vi "Main_01a.vi"() -> ()   [LabVIEW 2024]
panel:
  out "Right List":i32[](array[numeric])
  out "Left List":i32[](array[numeric])
  out "Answer 2344935":i32
  in  "Puzzle":string="80421   40193\n69841   31045\n47850   64065\n63141   52072\n32908   83033\n33395   25559\n78513   59127\n91270   76329\n65508   34159\n27139   15788\n13228   50396\n43186   29116\n55392   52441\n19309   68909\n72798   54258\n31590   11220\n32125   81946\n58099   50396\n16614   76682\n60604   12184\n21251   26105\n56053   96112\n47903   13396\n72956   11681\n66315   11220\n54499   96112\n38390   83884\n69211   52732\n69235   52441\n83831   49092\n25782   75523\n35417   15162\n45889   82918\n76191   97182\n95942   49643\n30121   83884\n86470   16217\n23572   11220\n69703   80739\n45792   21543\n76682   70230\n79585   83884\n64501   69361\n55546   92076\n43632   87826\n93309   17223\n73996   69071\n83466   42385\n73963   19398\n36643   98070\n43789   15788\n54302   70897\n83362   50227\n60881   66983\n61881   17864\n81520   52171\n99147   41180\n63427   16217\n50290   40193\n19315   20520\n84997   27666\n45495   40509\n81512   76682\n93459   11220\n28126   72353\n38227   11681\n49613   27677\n26858   40193\n16759   51946\n42145   90200\n64421   88733\n97361   16019\n32616   75596\n30875   90149\n82019   50759\n90554   83033\n42030   75763\n64459   32394\n45152   83884\n51375   48768\n71487   93793\n69694   84439\n97213   70998\n65471   90900\n69237   48307\n50672   58376\n61500   58064\n22831   76682\n63626   90356\n43195   87826\n67468   11770\n59753   97698\n34386   97698\n84851   23296\n96001   69910\n41418   13027\n82815   27666\n37012   17864\n45122   57830\n81552   44943\n18717   33011\n28726   87826\n29453   52441\n82398   24963\n47384   87826\n24205   50966\n80001   43568\n17033   21145\n74890   54233\n59065   58047\n33505   96112\n96403   34213\n35992   94345\n74353   27666\n59539   37101\n90355   71860\n86007   11220\n50733   76682\n75113   94664\n56735   87038\n27654   16492\n39478   47633\n70998   95331\n19885   38941\n47463   26105\n74771   28343\n56762   87773\n89980   35218\n35434   71473\n97275   53382\n97389   28343\n55060   11220\n83189   74164\n65464   75140\n15091   58376\n49752   94345\n55978   50227\n13991   40193\n58778   69071\n99285   16217\n37693   40193\n61282   71473\n34624   87374\n53881   13912\n67666   58376\n51235   52441\n80739   99593\n40193   97698\n94214   83205\n13145   72473\n88888   40193\n46957   96567\n92406   59738\n85389   13942\n55969   52441\n91426   46497\n92608   63775\n71473   24823\n51744   50396\n77645   42696\n34121   96112\n99775   96112\n89480   98660\n42647   95861\n35131   98522\n22031   76805\n10282   43806\n82323   65743\n79408   89179\n50692   85420\n89878   70998\n46431   17223\n99643   52441\n61276   68075\n14058   83884\n94292   17411\n92506   40193\n91012   17223\n51557   55254\n50846   96567\n20336   84821\n71617   81946\n40314   84439\n42990   89703\n62455   27446\n65790   94345\n57568   65105\n13052   79090\n30028   96128\n42028   58852\n47372   87826\n44459   90200\n67988   66776\n28313   84439\n52545   94345\n17108   37412\n16113   11681\n56064   54165\n60025   37314\n85545   11681\n68437   25575\n46677   20626\n53308   28343\n79483   70998\n54308   55727\n26755   69337\n73791   50227\n33565   83884\n35359   17223\n47840   26266\n50109   75074\n88842   39316\n84439   97698\n86029   96112\n39964   79122\n37828   69071\n73120   96567\n67688   50227\n61996   70230\n62643   82883\n99604   28343\n18054   76682\n52441   97698\n45131   58376\n32102   53380\n60963   53418\n73803   41652\n56361   70998\n74041   77517\n14940   84439\n80439   26105\n79199   83033\n41700   83033\n35229   65677\n64958   84439\n51246   78550\n23506   31244\n26237   40038\n49105   27712\n62117   37779\n76884   94345\n56414   62009\n88424   80739\n97192   15788\n70374   59226\n53515   76682\n85931   28343\n50925   38390\n51959   96567\n98082   28525\n37588   29342\n52624   37871\n28331   16217\n73762   94345\n73815   38390\n38573   25210\n88916   97698\n66917   28343\n47055   73500\n97902   34391\n16580   82128\n18015   91780\n77218   14792\n22251   37702\n62344   94345\n49811   73150\n43220   58572\n93889   76682\n70259   90173\n16985   26105\n93371   50227\n93434   49229\n97412   55737\n69071   39598\n70682   90271\n31536   30421\n81650   96112\n66094   70998\n94447   83052\n70230   87681\n69613   93387\n50227   85660\n32751   83903\n12441   41367\n64171   79090\n88431   75578\n33033   96567\n96305   79090\n17193   52441\n42766   27666\n30798   50396\n18160   14792\n86048   69517\n26894   10883\n72243   38390\n48910   96875\n80507   90612\n77344   83033\n11713   96112\n36810   50227\n91347   11220\n20755   76682\n50353   95421\n63754   63013\n22119   25388\n35010   38390\n39083   90678\n16379   13640\n47651   67154\n50798   71473\n64108   83884\n62368   85420\n87732   54461\n44496   74078\n50396   16217\n32142   94345\n12969   50227\n63851   24208\n59124   89844\n24929   21174\n55229   84439\n78807   15788\n58298   50396\n16926   96567\n83884   50396\n63542   49739\n76625   41626\n97382   32976\n40464   38390\n14575   10840\n63334   71473\n25579   40921\n71524   96567\n50616   93389\n81504   17864\n10618   32838\n65653   11681\n74217   76682\n17739   45245\n12975   56728\n92629   12987\n13610   68591\n24487   83033\n12475   81946\n31651   39134\n32359   81946\n41174   79359\n63548   65603\n55031   50396\n59183   58376\n74036   69252\n33977   71473\n39977   40407\n32033   40193\n90147   83033\n23940   30137\n67597   33156\n64295   99755\n72689   96112\n92379   83884\n59904   17864\n59250   54829\n31693   34134\n88853   97698\n46754   31254\n58208   11220\n98626   11220\n46741   70998\n36408   63013\n18581   87826\n63114   28343\n97394   81946\n93270   97698\n80744   59372\n97689   57651\n87482   58376\n11896   75807\n65025   96196\n15892   54686\n68939   24270\n16022   53606\n36023   85420\n95998   43637\n61265   38390\n79090   11220\n81946   99814\n63895   78782\n83527   90200\n51915   62980\n22548   20223\n58376   26608\n81705   24971\n99116   26106\n92178   77949\n98976   38390\n81016   28343\n52646   79090\n29911   88246\n23834   92181\n46484   89669\n68488   44503\n74484   29808\n89780   86262\n96112   75203\n51392   42994\n19800   23307\n49890   41317\n98098   94345\n57894   69730\n59120   93793\n86825   83884\n41981   84710\n69860   70998\n25576   35489\n42850   23083\n34439   85430\n91153   35450\n59806   16217\n87651   74318\n15466   76682\n94237   22001\n45392   47159\n35295   95111\n86122   88173\n28631   50396\n34798   26613\n61839   13468\n61723   96112\n14034   96112\n30006   16217\n14649   26145\n86294   80739\n32258   11681\n92857   50396\n86334   58376\n10895   84439\n63194   85936\n76887   96027\n68733   26105\n41207   63013\n28365   88512\n24732   38390\n67548   49710\n81155   48747\n41815   96112\n51642   69071\n62718   81572\n59606   98715\n74964   13588\n64466   17223\n96982   46340\n84527   94623\n69698   11220\n11144   23375\n57947   97698\n41007   80545\n11681   32334\n94807   43967\n54555   94345\n16363   93419\n65623   45980\n42388   45727\n48482   79090\n85324   81581\n59768   37611\n62042   11681\n90240   19425\n66983   24278\n98892   42679\n35839   35139\n17825   39236\n74183   28343\n94347   48434\n82766   84797\n12488   62200\n11529   58265\n82862   27666\n63390   87826\n87638   60767\n69964   71473\n94668   76682\n58958   52441\n75722   97743\n68139   11220\n58242   75810\n92586   40193\n29680   94345\n33347   73583\n74149   73747\n88092   94345\n82865   45901\n88894   38390\n40872   97309\n85420   93793\n80641   69071\n57680   79788\n50575   63583\n45838   28855\n77834   63196\n36094   58852\n93487   19648\n98316   79122\n89283   97494\n81283   78824\n78086   84439\n70708   27959\n64643   44369\n39933   56445\n68663   28343\n97698   10803\n79122   51608\n35053   96112\n88445   87826\n59362   81946\n58091   67264\n48218   93793\n64495   16994\n38395   71473\n61884   50396\n84809   84439\n90363   78607\n39707   76682\n66866   83033\n76807   80277\n98492   83033\n65436   84059\n69199   68798\n62230   83884\n51938   18013\n99036   22915\n20508   84439\n41393   50396\n47979   58852\n74140   70998\n42029   88646\n43056   14163\n96145   39532\n80632   64382\n56985   85420\n63903   41993\n11220   93712\n94345   15788\n43760   56901\n93453   58852\n35914   74746\n73054   44762\n45629   40193\n77231   55896\n77041   38390\n96658   74157\n46466   17606\n88020   77476\n51115   61806\n24234   81946\n17382   79090\n38939   78416\n55399   95124\n74933   97972\n17223   11832\n20126   25792\n84054   91443\n84057   96112\n88765   83033\n27933   54577\n48695   78824\n90200   51999\n74599   38503\n61441   90200\n66742   38390\n23353   26105\n37362   82425\n38602   44514\n41407   71473\n51001   62633\n98321   40630\n75078   11681\n68245   24288\n49051   14363\n36869   25312\n17659   47253\n74211   69071\n41285   22997\n89913   71473\n35951   34861\n67158   50396\n43938   15553\n72373   24972\n40926   97698\n63013   85420\n19477   71473\n79722   19841\n28842   83920\n14541   55730\n31500   75763\n51488   32218\n18889   96567\n57241   17864\n51819   47021\n21973   30568\n13743   10104\n87695   43875\n90862   27666\n16780   65150\n24792   58376\n28715   69071\n40287   78011\n59897   84439\n16124   83884\n34237   44208\n80709   83186\n12989   55204\n96071   63816\n78189   63337\n37586   98216\n19413   51370\n64986   70521\n93855   48927\n57998   25233\n42676   58360\n93905   29575\n18012   58243\n28846   54313\n97083   50396\n59982   20815\n95409   88260\n57482   70230\n69515   83884\n78295   69071\n72645   71473\n71966   28343\n98274   84439\n34068   28343\n96135   40193\n65836   15788\n23264   84439\n19621   51691\n75945   40091\n29573   47799\n14879   79090\n28207   38390\n11483   15774\n32877   80739\n36254   96567\n65116   27258\n14250   93650\n23902   96112\n89984   35958\n82242   33004\n12762   62900\n81194   99347\n72193   37712\n71644   74162\n46588   52441\n27739   70311\n35648   70998\n44410   87233\n46656   27666\n31914   71473\n90034   78824\n61968   83033\n36567   29131\n78387   67697\n33453   57266\n24915   40540\n70857   52975\n28343   81423\n92106   87378\n56025   82509\n32851   98692\n51436   97147\n70601   71473\n70452   33153\n39288   15788\n17976   11220\n15788   58376\n40113   53779\n25192   88120\n31980   98924\n80317   91384\n67936   10228\n14839   75691\n55689   75265\n28107   90207\n49283   17864\n27666   52539\n26105   26025\n71897   10363\n65171   58095\n87061   76361\n58586   84439\n90319   17223\n12401   11681\n60665   21206\n66454   77367\n58801   69471\n12007   11220\n59620   71043\n14269   33941\n84020   34182\n21849   61119\n19934   93793\n49226   64719\n59477   58376\n67180   38390\n69143   84212\n29611   69071\n74186   73216\n44892   47027\n88341   63662\n93425   27666\n58009   40217\n61426   88678\n14176   17223\n19374   19815\n15924   63644\n31338   90200\n20061   96567\n77739   17223\n39213   79090\n86112   44465\n59347   96112\n52900   88643\n49030   41964\n79160   96112\n60822   33345\n87682   46340\n92223   67780\n75763   68868\n58470   38390\n22344   11681\n60094   70230\n53703   65992\n60348   41120\n14792   81993\n53271   21427\n67055   17864\n64402   49401\n46340   71473\n67425   80739\n33676   91364\n20261   93934\n33464   45079\n47333   87047\n99552   33828\n46700   29241\n34066   38390\n63635   81946\n64943   90200\n93222   70855\n39852   27666\n54215   27846\n91837   81435\n13206   92486\n34097   89083\n67571   63013\n65552   28794\n93206   16217\n57258   46746\n12355   95783\n45193   39825\n78824   41374\n79640   28343\n33304   46968\n52405   53684\n80165   79090\n63764   98552\n50867   62235\n55169   67322\n17385   63412\n93847   84439\n86220   96567\n56922   26105\n93793   70998\n46061   15119\n60608   50227\n53721   82034\n37048   97113\n78634   17392\n16149   11220\n96567   17864\n67761   15242\n43531   45273\n28649   81808\n16807   11681\n35016   38390\n36328   15788\n47350   87826\n83703   76682\n96035   68596\n89445   40193\n39175   22115\n46972   69071\n86512   64757\n70145   30941\n92472   94345\n28607   84439\n97839   80739\n46293   22854\n39471   56487\n40895   81224\n79054   15540\n19112   99099\n87456   97698\n64947   93293\n46868   17223\n61194   51103\n94011   51317\n93446   67760\n51603   79090\n98462   32618\n87627   14792\n50434   28343\n80823   87826\n85968   11220\n70582   94611\n69082   69071\n82872   75587\n66992   93001\n16652   81390\n45397   67124\n48288   12534\n16683   60958\n28845   17300\n73108   85770\n10887   14000\n86564   58432\n73753   15788\n58200   60971\n14724   10521\n22429   86503\n15636   73714\n42007   50396\n83033   28343\n11018   17864\n84668   59520\n34407   50227\n21979   66729\n20788   97698\n88249   71473\n29698   76682\n18861   90200\n33097   18831\n84374   38460\n42337   49469\n96184   11220\n93246   50708\n59059   17223\n94799   11681\n94592   90061\n16217   87826\n15119   39287\n98585   71473\n96536   42853\n70453   24363\n98772   69071\n86608   28722\n96532   50396\n29434   83821\n45190   18432\n39085   52441\n14544   27666\n98167   83884\n40247   35796\n58852   95208\n63594   94345\n37166   70696\n37060   97185\n78269   17223\n31684   50764\n17864   52599\n24791   33385\n88009   94208\n44960   66939\n94307   25038\n97941   92450\n84015   83884\n18910   52086\n65496   17223\n40031   34551\n85606   91632\n61769   76682\n16593   90387\n18746   84938\n37661   78508\n74488   71473\n10696   57789\n73457   33795\n36702   93793\n50523   40193\n54560   97491\n31840   38390\n76940   40193\n16870   11681\n59273   30259\n87826   11069\n42351   47872\n46704   17864\n60979   83884\n13487   66385\n89414   94345\n95781   78824\n81388   50396\n76147   16961\n47912   27666\n38794   15498\n42095   60345\n50754   85082\n47680   11681\n74650   63013\n79979   27666\n93963   91067\n12526   51125\n15421   50227\n14489   17864\n19890   71473\n39148   69071\n35061   43580\n13873   78824\n65002   84439\n44196   70230\n91160   27666\n66243   17864\n68520   52987\n57313   11001\n97451   71232\n45491   88748\n72806   28343\n10935   96112\n26571   50227\n36588   11220\n97082   47405\n74083   76682\n13709   28343\n71565   60347\n67060   89690\n89812   68984\n64357   18200\n13576   86923\n17785   52441\n90523   87826\n48169   84439\n49404   96112\n38548   93793\n10365   50396\n85079   97698\n87583   95586\n63995   97698\n37765   62288\n96507   26105\n74440   19405\n96601   94432\n37066   38390\n42143   11552\n33431   27666\n77502   63356\n33810   52441\n14847   36105\n21823   66983\n57868   71473\n84231   27666\n87717   52441\n53162   97698\n35374   65715\n34570   26105\n20224   36282\n71791   40193\n18833   48330\n12194   83762\n92449   38390\n18772   71473\n59035   57762\n60408   76682\n62373   63013\n79934   40193\n82312   59106\n22944   72620\n15001   50192\n42041   93793\n27226   80739\n68012   30136\n22148   34448\n15624   94345\n79255   39850\n80907   18558\n92896   15318\n25411   94345\n33580   81946\n71575   70650\n47700   79090\n75865   16217\n48756   81946\n98547   75763\n23220   38390\n15241   79090\n18586   33917\n22280   40494\n35998   69327\n60853   95280\n38251   50396\n52525   87826"
  in  "Example":string="3   4\n4   3\n2   5\n1   3\n3   9\n3   3"
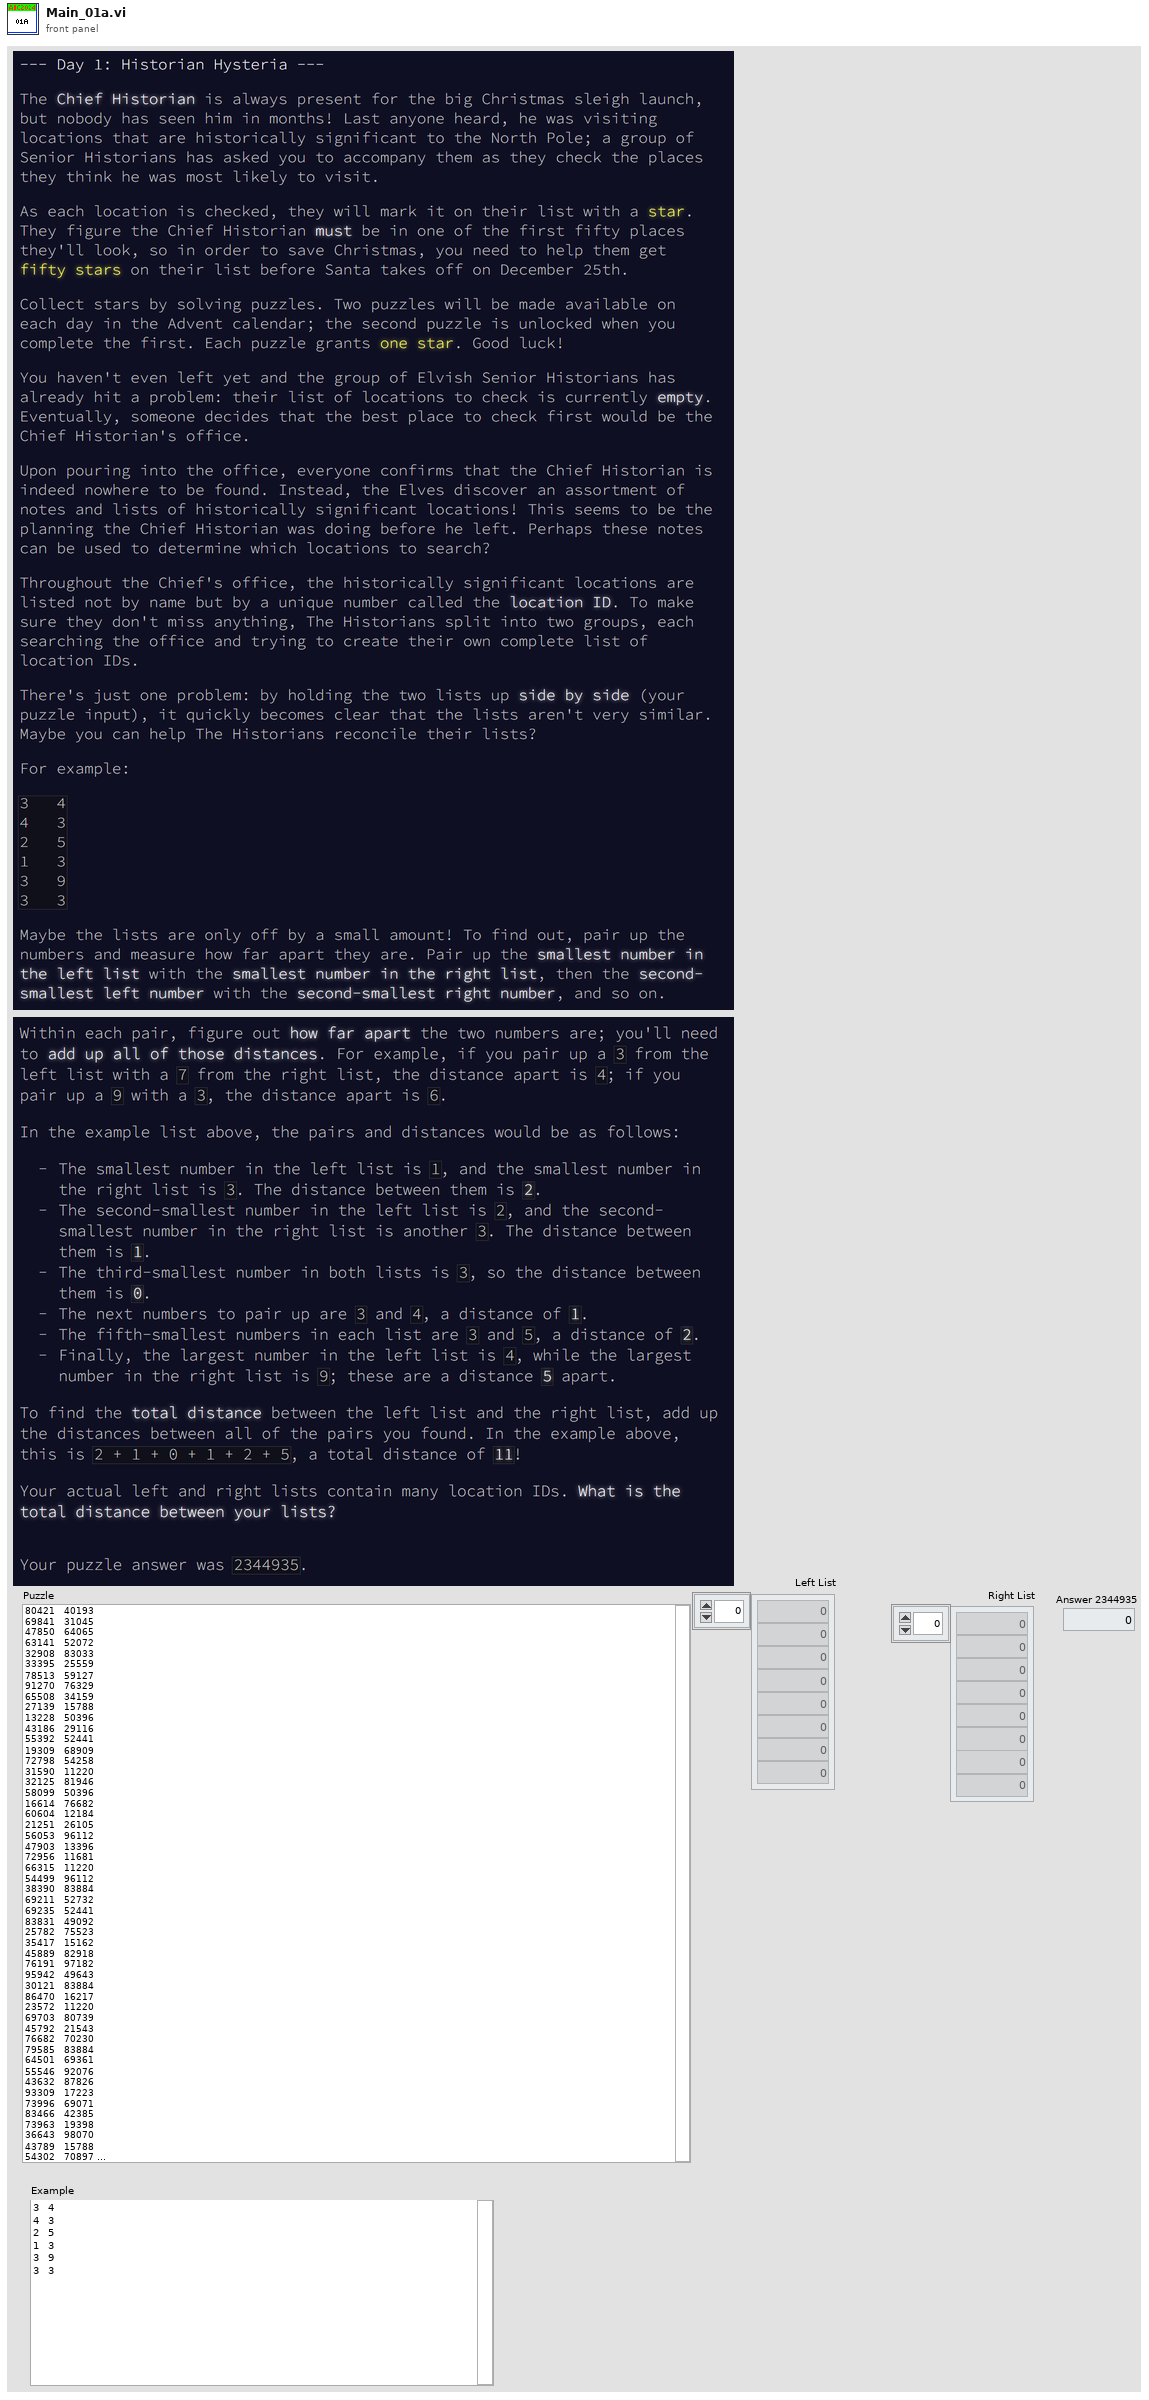
[diagram p1: front panel]
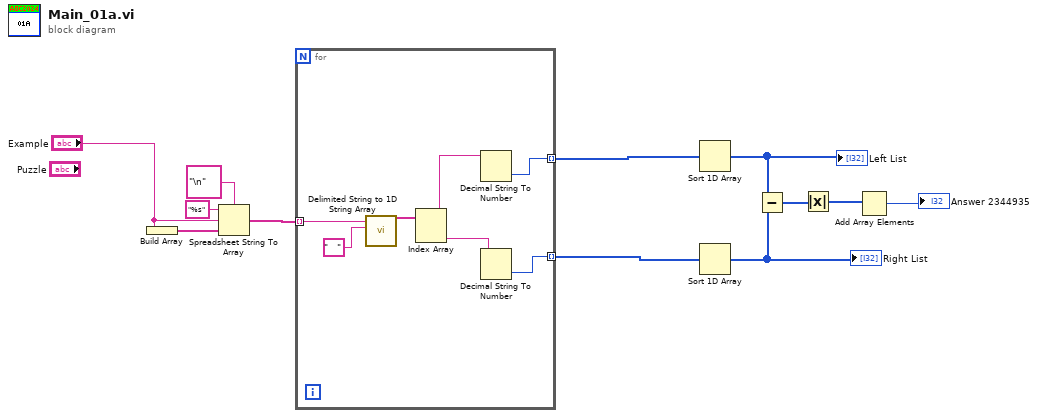
[diagram p0: block diagram]
diagram:
  n1 = Build Array("Example") -> (w12:string[])
  n2 = Spreadsheet String To Array(delimiter (Tab)="\n", format string="%s", spreadsheet string="Example", array type (2D Dbl)=w12) -> (array=w9:string[])
  n3 = for {
    tunnel: w9 -> [w19] mode=indexing
    tunnel: [w14] -> w8 mode=indexing
    tunnel: [w13] -> w7 mode=indexing
    n4 = call <vilib>:"Delimited String to 1D String Array.vi"("delimiter"="   ", "delimited string"=w19) -> ("string array"=w18:string[])  [unwired: 9 in]
    n5 = Index Array(array=w18) -> (element #1=w17:string, element #2=w16:string)  [unwired: 2 in]
    n6 = Decimal String To Number(string=w17) -> (number=w14:i32)  [unwired: 2 in, 1 out]
    n7 = Decimal String To Number(string=w16) -> (number=w13:i32)  [unwired: 2 in, 1 out]
  }
  n8 = Sort 1D Array(array=w8) -> (sorted array=w6:i32[])
  "Left List" <- w6
  n9 = Sort 1D Array(array=w7) -> (sorted array=w5:i32[])
  "Right List" <- w5
  n10 = Subtract(x=w6, y=w5) -> (x-y=w4:i32[])
  n11 = Absolute Value(x=w4) -> (abs(x)=w3:i32[])
  n12 = Add Array Elements(numeric array=w3) -> (sum=→"Answer 2344935":i32)
